vi "fpga_output.vi"(4 "limit (high, 10 V)":T1, 5 "slope":cluster{"x":sgl, "y":sgl}, 6 "limit (low, 10 V)":T1, 7 "gain":T1, 11 "output (in)":T1) -> (2 "inrange?":bool, 3 "output (out)":T1)   [LabVIEW 2021]
doc: "Output the values.\n\nThe output will converted with gain (AO = output / gain) and limited with \"limit (low, 10 V)\" and \"limit (high, 10 V)\"."
uses:
  fpga_dtype_sgl_8ch.ctl
  <vilib>/rvi/eio/common/nirviEmuTemplateMethod_errors.vi
  <vilib>/eio/EIONode/EIONode.xnode
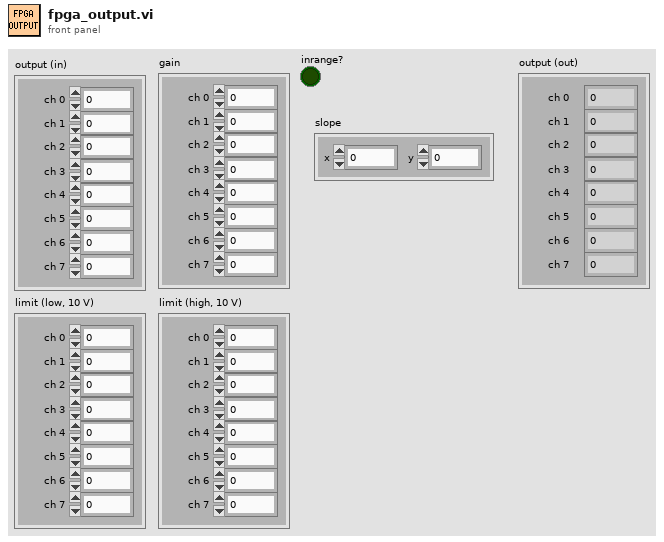
[diagram p1: front panel]
types:
  T1 = typedef "fpga_dtype_sgl_8ch.ctl" = cluster{"ch 0":sgl, "ch 1":sgl, "ch 2":sgl, "ch 3":sgl, "ch 4":sgl, "ch 5":sgl, "ch 6":sgl, "ch 7":sgl}
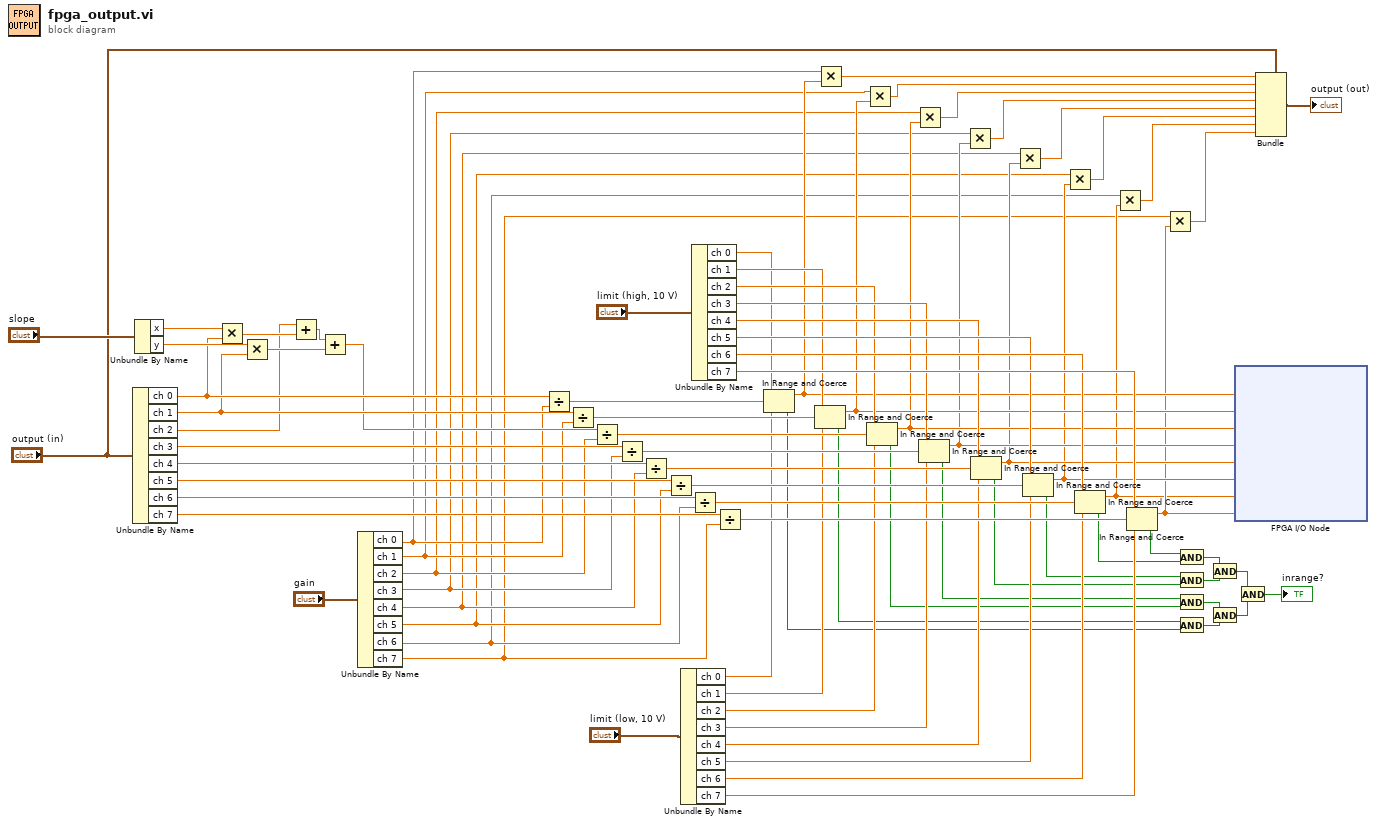
[diagram p0: block diagram]
diagram:
  n1 = Unbundle By Name("output (in)") -> ("ch 0"=w33:sgl, "ch 1"=w32:sgl, "ch 2"=w28:sgl, "ch 3"=w81:sgl, "ch 4"=w80:sgl, "ch 5"=w79:sgl, "ch 6"=w78:sgl, "ch 7"=w82:sgl)
  n2 = Unbundle By Name("slope") -> ("x"=w35:sgl, "y"=w34:sgl)
  n3 = Multiply(x=w35, y=w33) -> (x*y=w29:sgl)
  n4 = Multiply(x=w34, y=w32) -> (x*y=w31:sgl)
  n5 = Add(x=w28, y=w29) -> (x+y=w30:sgl)
  n6 = Add(x=w30, y=w31) -> (x+y=w27:sgl)
  n7 = Unbundle By Name("gain") -> ("ch 0"=w18:sgl, "ch 1"=w17:sgl, "ch 2"=w16:sgl, "ch 3"=w15:sgl, "ch 4"=w14:sgl, "ch 5"=w13:sgl, "ch 6"=w12:sgl, "ch 7"=w11:sgl)
  n8 = Divide(x=w33, y=w18) -> (x/y=w77:sgl)
  n9 = Divide(x=w32, y=w17) -> (x/y=w70:sgl)
  n10 = Divide(x=w27, y=w16) -> (x/y=w71:sgl)
  n11 = Divide(x=w81, y=w15) -> (x/y=w72:sgl)
  n12 = Divide(x=w80, y=w14) -> (x/y=w73:sgl)
  n13 = Divide(x=w79, y=w13) -> (x/y=w74:sgl)
  n14 = Unbundle By Name("limit (low, 10 V)") -> ("ch 0"=w59:sgl, "ch 1"=w58:sgl, "ch 2"=w57:sgl, "ch 3"=w56:sgl, "ch 4"=w55:sgl, "ch 5"=w54:sgl, "ch 6"=w53:sgl, "ch 7"=w52:sgl)
  n15 = Divide(x=w78, y=w12) -> (x/y=w75:sgl)
  n16 = Unbundle By Name("limit (high, 10 V)") -> ("ch 0"=w60:sgl, "ch 1"=w61:sgl, "ch 2"=w62:sgl, "ch 3"=w63:sgl, "ch 4"=w64:sgl, "ch 5"=w65:sgl, "ch 6"=w66:sgl, "ch 7"=w67:sgl)
  n17 = Divide(x=w82, y=w11) -> (x/y=w76:sgl)
  n18 = In Range and Coerce(upper limit=w60, x=w77, lower limit=w59) -> (coerced(x)=w26:sgl, In Range?=w44:bool)
  n19 = In Range and Coerce(upper limit=w61, x=w70, lower limit=w58) -> (coerced(x)=w25:sgl, In Range?=w45:bool)
  n20 = Multiply(x=w18, y=w26) -> (x*y=w10:sgl)
  n21 = Multiply(x=w17, y=w25) -> (x*y=w9:sgl)
  n22 = In Range and Coerce(upper limit=w62, x=w71, lower limit=w57) -> (coerced(x)=w24:sgl, In Range?=w46:bool)
  n23 = Multiply(x=w16, y=w24) -> (x*y=w8:sgl)
  n24 = In Range and Coerce(upper limit=w63, x=w72, lower limit=w56) -> (coerced(x)=w23:sgl, In Range?=w47:bool)
  n25 = Multiply(x=w15, y=w23) -> (x*y=w7:sgl)
  n26 = In Range and Coerce(upper limit=w64, x=w73, lower limit=w55) -> (coerced(x)=w22:sgl, In Range?=w48:bool)
  n27 = Multiply(x=w14, y=w22) -> (x*y=w6:sgl)
  n28 = In Range and Coerce(upper limit=w65, x=w74, lower limit=w54) -> (coerced(x)=w21:sgl, In Range?=w49:bool)
  n29 = Multiply(x=w13, y=w21) -> (x*y=w5:sgl)
  n30 = In Range and Coerce(upper limit=w66, x=w75, lower limit=w53) -> (coerced(x)=w19:sgl, In Range?=w50:bool)
  n31 = Multiply(x=w12, y=w19) -> (x*y=w4:sgl)
  n32 = In Range and Coerce(upper limit=w67, x=w76, lower limit=w52) -> (coerced(x)=w20:sgl, In Range?=w51:bool)
  n33 = Multiply(x=w11, y=w20) -> (x*y=w3:sgl)
  n34 = And(x=w51, y=w50) -> (x .and. y?=w40:bool)
  n35 = And(x=w49, y=w48) -> (x .and. y?=w41:bool)
  n36 = And(x=w47, y=w46) -> (x .and. y?=w42:bool)
  n37 = And(x=w45, y=w44) -> (x .and. y?=w43:bool)
  n38 = And(x=w40, y=w41) -> (x .and. y?=w38:bool)
  n39 = And(x=w42, y=w43) -> (x .and. y?=w39:bool)
  n40 = xnode "FPGA I/O Node"("Connector0/AO0"=w26, "Connector0/AO1"=w25, "Connector0/AO2"=w24, "Connector0/AO3"=w23, "Connector0/AO4"=w22, "Connector0/AO5"=w21, "Connector0/AO6"=w19, "Connector0/AO7"=w20) -> ()  [unwired: 8 in, 8 out]
  n41 = And(x=w38, y=w39) -> (x .and. y?=→"inrange?":bool)
  n42 = Bundle(cluster="output (in)", "ch 0"=w10, "ch 1"=w9, "ch 2"=w8, "ch 3"=w7, "ch 4"=w6, "ch 5"=w5, "ch 6"=w4, "ch 7"=w3) -> (→"output (out)":T1)
